vi "Write Key (I32).vi"(7 "section":string, 8 "error in (no error)":errorcluster, 9 "value":i32, 10 "key":string, 11 "refnum":T1) -> (0 "error out":errorcluster, 3 "refnum out":T1)   [LabVIEW 2009]
doc: "Writes a value to a key in a specified section of the configuration data identified by <B>refnum</B>. You can use this polymorphic VI to write Boolean, double-precision numeric, signed integer, path, string, or unsigned integer values to a key. The data type you wire to the <B>value</B> input determines the polymorphic instance to use."
uses:
  <vilib>/Utility/config.llb/Config Data RefNum.ctl
  Config Data Modify Functions.ctl
  <vilib>/Utility/config.llb/NI_LVConfig.lvlib
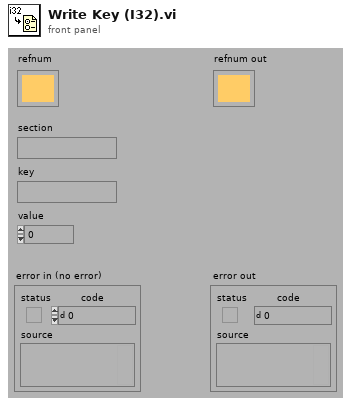
[diagram p1: front panel]
types:
  T1 = typedef "NI_LVConfig.lvlib/Config Data RefNum.ctl" = refnum<k1>
  T2 = typedef "Config Data Modify Functions.ctl" = enum16{"set file path", "put data", "add key", "remove section", "remove key"}
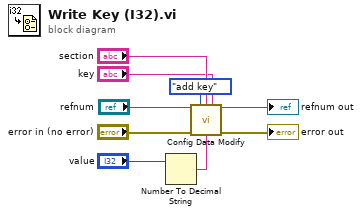
[diagram p0: block diagram]
diagram:
  n1 = Number To Decimal String(number="value") -> (decimal integer string=w3:string)  [unwired: 1 in]
  n2 = call "Config Data Modify.vi"("config data"="refnum", "function"=Config_Data_Modify_Functions."add key", "section"="section", "key"="key", "error in (no error)"="error in (no error)", "value"=w3) -> ("config data out"=→"refnum out":T1, "error out"=→"error out":errorcluster)  [unwired: 6 in, 2 out]
